vi "Plot Spectrum.vi"(0 "Optical Spectrum Plot":T1, 5 "Optical Spectrum":enum32{"Energy", "Wavelength", "Raman Shift"}(tab), 7 "Spectrum":T2, 11 "error in (no error)":errorcluster, 12 "Update Pane?":bool) -> (4 "Optical Spectrum vs Energy":cluster{"data":dbl[], "data":dbl[]}(graph), 6 "Optical Spectrum vs Wavelength":cluster{"data":dbl[], "data":dbl[]}(graph), 8 "Optical Spectrum vs Raman Shift":cluster{"data":dbl[], "data":dbl[]}(graph), 15 "error out":errorcluster)   [LabVIEW 2014]
uses:
  Hardware Control/Spectrometer/Spectral Data.ctl
  Optical Spectrum Plot Refnum.ctl
panel:
  out "Detector Temperature":dbl
  # "LICENSED MATERIALS – PROPERTY OF IBM\nCopyright IBM Corp. 2016,\nALL RIGHTS RESERVED"
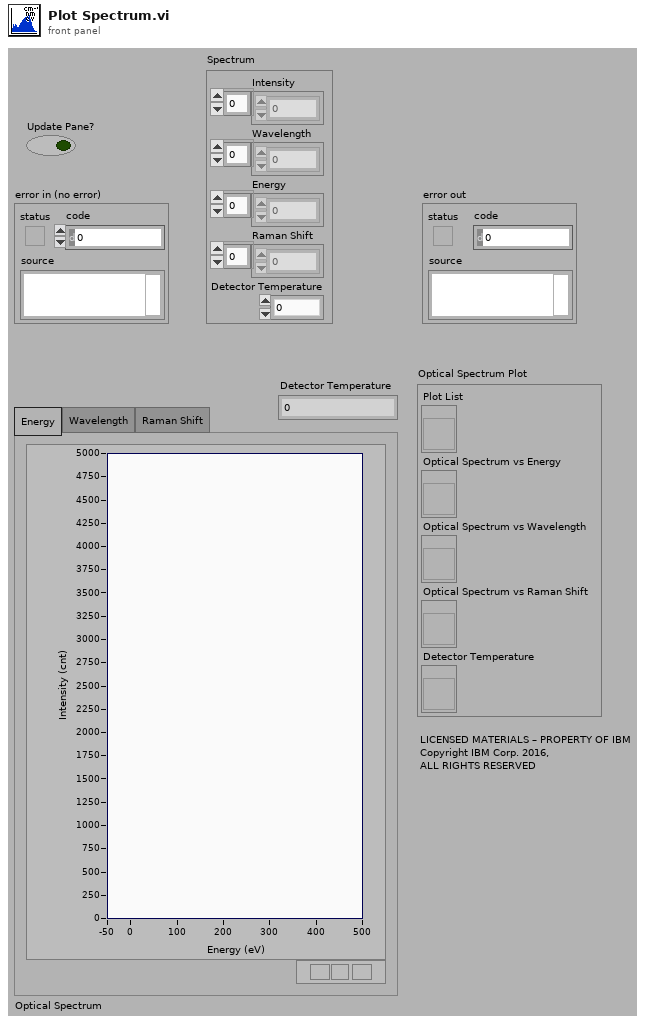
[diagram p1: front panel]
types:
  T1 = typedef "Optical Spectrum Plot Refnum.ctl" = cluster{"Plot List":refnum<vi>, "Optical Spectrum vs Energy":refnum<vi>, "Optical Spectrum vs Wavelength":refnum<vi>, "Optical Spectrum vs Raman Shift":refnum<vi>, "Detector Temperature":refnum<vi>}
  T2 = typedef "Spectral Data.ctl" = cluster{"Intensity":dbl[], "Wavelength":dbl[], "Energy":dbl[], "Raman Shift":dbl[], "Detector Temperature":dbl}
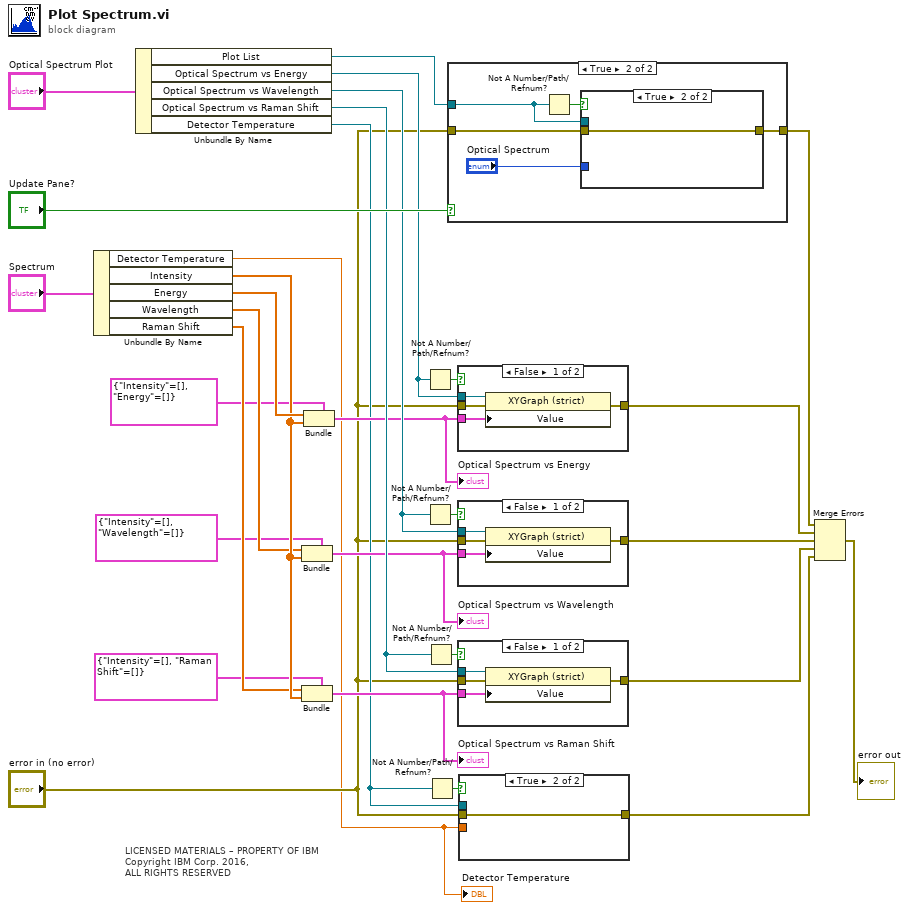
[diagram p0: block diagram]
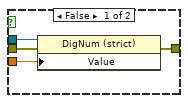
[diagram p2: hidden frame]
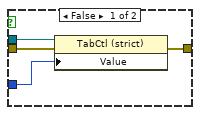
[diagram p4: hidden frame]
diagram:
  # "LICENSED MATERIALS – PROPERTY OF IBM\nCopyright IBM Corp. 2016,\nALL RIGHTS RESERVED"
  n1 = Unbundle By Name("Spectrum") -> ("Detector Temperature"=w1:dbl, "Intensity"=w26:dbl[], "Energy"=w29:dbl[], "Wavelength"=w25:dbl[], "Raman Shift"=w24:dbl[])
  "Detector Temperature" <- w1
  n2 = Unbundle By Name("Optical Spectrum Plot") -> ("Plot List"=w17:refnum<vi>, "Optical Spectrum vs Energy"=w13:refnum<vi>, "Optical Spectrum vs Wavelength"=w14:refnum<vi>, "Optical Spectrum vs Raman Shift"=w15:refnum<vi>, "Detector Temperature"=w4:refnum<vi>)
  n3 = Bundle(cluster=cluster{"Intensity":dbl[], "Wavelength":dbl[]} {"Intensity"=[], "Wavelength"=[]} ("Optical Spectrum vs Energy 2"), "Intensity"=w25, "Wavelength"=w26) -> (w11:cluster{"Intensity":dbl[], "Wavelength":dbl[]})
  "Optical Spectrum vs Wavelength" <- w11
  n4 = Bundle(cluster=cluster{"Intensity":dbl[], "Raman Shift":dbl[]} {"Intensity"=[], "Raman Shift"=[]} ("Optical Spectrum vs Energy 2"), "Intensity"=w24, "Raman Shift"=w26) -> (w10:cluster{"Intensity":dbl[], "Raman Shift":dbl[]})
  "Optical Spectrum vs Raman Shift" <- w10
  n5 = Bundle(cluster=cluster{"Intensity":dbl[], "Energy":dbl[]} {"Intensity"=[], "Energy"=[]} ("Optical Spectrum vs Energy 2"), "Intensity"=w29, "Energy"=w26) -> (w12:cluster{"Intensity":dbl[], "Energy":dbl[]})
  "Optical Spectrum vs Energy" <- w12
  n6 = Not A Number/Path/Refnum?(number/path/refnum=w13) -> (NaN/Path/Refnum?=w23:bool)
  n7 = Not A Number/Path/Refnum?(number/path/refnum=w14) -> (NaN/Path/Refnum?=w22:bool)
  n8 = Not A Number/Path/Refnum?(number/path/refnum=w15) -> (NaN/Path/Refnum?=w21:bool)
  n9 = Not A Number/Path/Refnum?(number/path/refnum=w4) -> (NaN/Path/Refnum?=w5:bool)
  n10 = case shown="True" "Update Pane?" {
    tunnel: [w31 w35] -> w9
    tunnel: w17 -> [_ w33]
    tunnel: "error in (no error)" -> [w31 w32]
    frame False {
    }
    frame True {
      n11 = Not A Number/Path/Refnum?(number/path/refnum=w33) -> (NaN/Path/Refnum?=w36:bool)
      n12 = case shown="True" w36 {
        tunnel: [w40 w41] -> w35
        tunnel: "Optical Spectrum" -> [w39 _]
        tunnel: w33 -> [w38 _]
        tunnel: w32 -> [w37 w41]
        frame False {
          n13 = property class="TabCtl (strict)"(reference=w38, error in=w37, "Value"=w39) -> (error out=w40:errorcluster)  [unwired: 1 out]
        }
        frame True {
        }
      }
    }
  }
  n14 = case shown="False" w23 {
    tunnel: "error in (no error)" -> [w45 w46]
    tunnel: [w44 w46] -> w20
    tunnel: w13 -> [w43 _]
    tunnel: w12 -> [w42 _]
    frame False {
      n15 = property class="XYGraph (strict)"(reference=w43, error in=w45, "Value"=w42) -> (error out=w44:errorcluster)  [unwired: 1 out]
    }
    frame True {
    }
  }
  n16 = case shown="False" w22 {
    tunnel: "error in (no error)" -> [w50 w51]
    tunnel: [w49 w51] -> w19
    tunnel: w14 -> [w48 _]
    tunnel: w11 -> [w47 _]
    frame False {
      n17 = property class="XYGraph (strict)"(reference=w48, error in=w50, "Value"=w47) -> (error out=w49:errorcluster)  [unwired: 1 out]
    }
    frame True {
    }
  }
  n18 = case shown="False" w21 {
    tunnel: "error in (no error)" -> [w55 w56]
    tunnel: [w54 w56] -> w18
    tunnel: w15 -> [w53 _]
    tunnel: w10 -> [w52 _]
    frame False {
      n19 = property class="XYGraph (strict)"(reference=w53, error in=w55, "Value"=w52) -> (error out=w54:errorcluster)  [unwired: 1 out]
    }
    frame True {
    }
  }
  n20 = case shown="True" w5 {
    tunnel: [w60 w61] -> w2
    tunnel: w4 -> [w59 _]
    tunnel: "error in (no error)" -> [w58 w61]
    tunnel: w1 -> [w57 _]
    frame False {
      n21 = property class="DigNum (strict)"(reference=w59, error in=w58, "Value"=w57) -> (error out=w60:errorcluster)  [unwired: 1 out]
    }
    frame True {
    }
  }
  n22 = Merge Errors(w9, w20, w19, w18, w2) -> (→"error out":errorcluster)
